vi "Initialization VI.vi"(8 "error in (no error)":errorcluster, 10 "Custom XML":string, 11 "Device Item Ref in":T1 format="%.0x") -> (0 "error out":errorcluster, 3 "Device Item Ref out":T1 format="%.0x")   [LabVIEW 2019, in "Protection and Counter Addon System Explorer.lvlib"]
uses:
  Protection and Counter Addon System Explorer.lvlib
  <vilib>/NI VeriStand/Custom Device API/Custom Device Item Ref.ctl
  <vilib>/NI VeriStand/Custom Device API/Custom Device Channel.ctl
  <vilib>/NI VeriStand/Custom Device API/Custom Device Channel Type.ctl
  Addon Shared/SubVIs/GUID Lookup.vi
  <vilib>/NI VeriStand/Custom Device API/Custom Device API.lvlib
  Addon Shared/Protection and Counter Addon Shared.lvlib
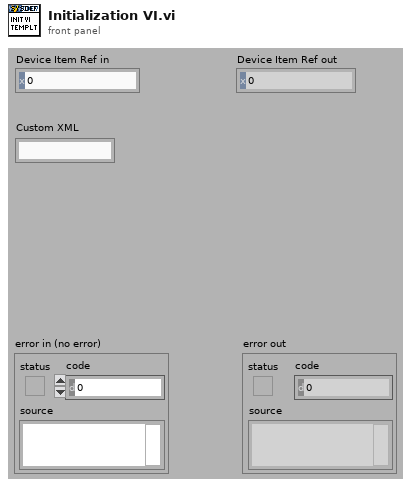
[diagram p1: front panel]
types:
  T1 = typedef "Custom Device API.lvlib/Custom Device Item Ref.ctl" = u64
  T2 = typedef "Custom Device API.lvlib/Custom Device Channel.ctl" = cluster{"Type":T3, "Units":string, "Default Value":dbl, "Faultable":bool, "Scalable":bool}
  T3 = typedef "Custom Device API.lvlib/Custom Device Channel Type.ctl" = enum16{"Input", "Output"}
  T4 = typedef "Protection and Counter Addon Shared.lvlib/XNET Settings.ctl" = cluster{"Database":refnum<k21>, "Cluster":refnum<k21>, "Port":string, "Baud rate [Bd]":u64, "Termination":u32, "CAN I/O Mode":u32, "FD Baud rate [Bd]":u64, "Priority":i32, "Use Legacy":bool}
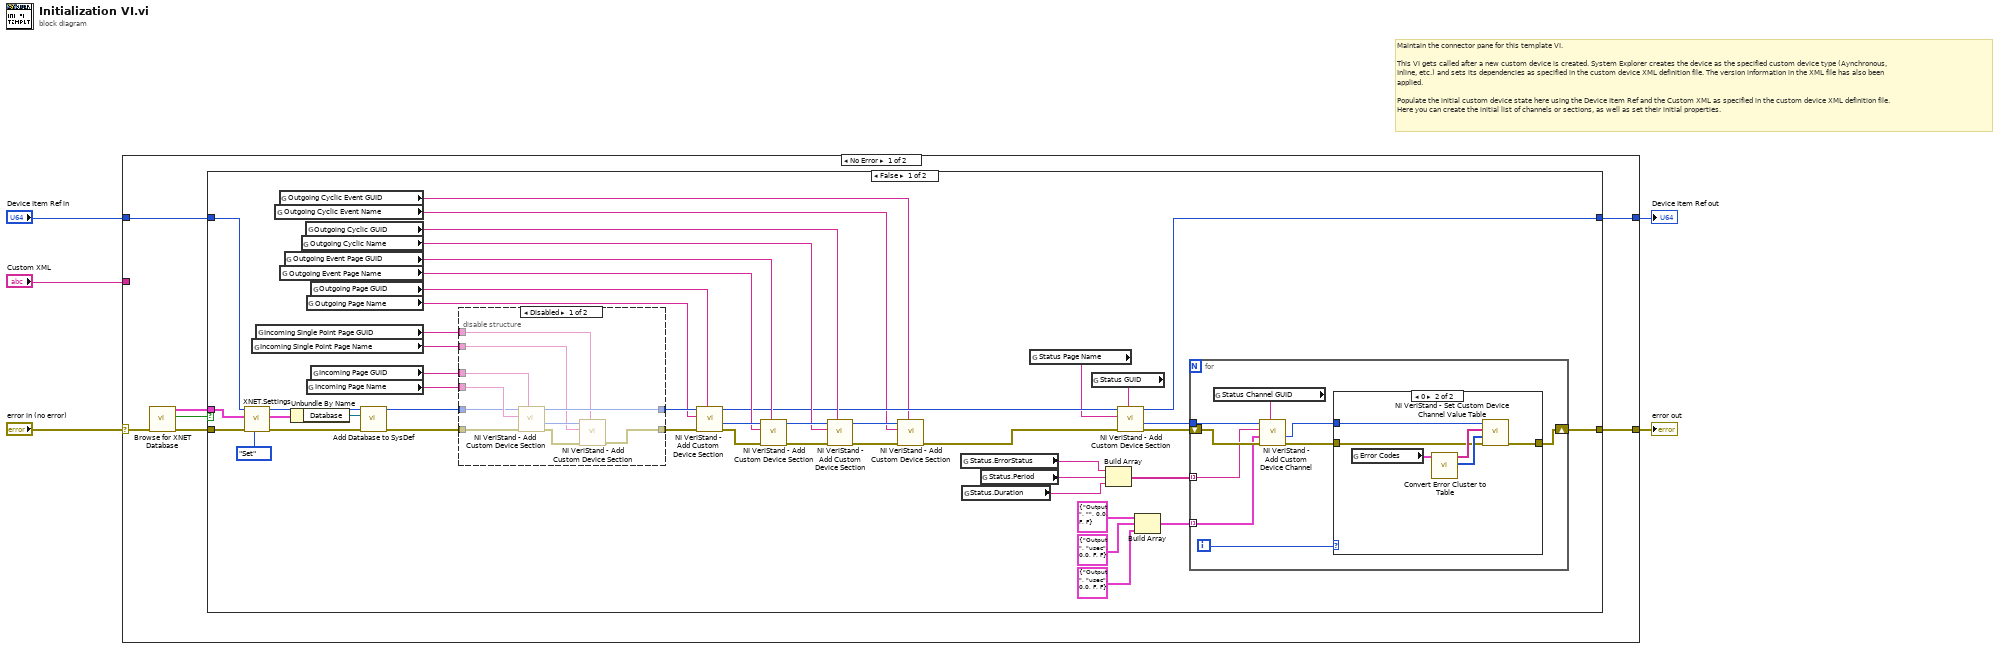
[diagram p0: block diagram]
diagram:
  # "Maintain the connector pane for this template VI.\n\nThis VI gets called after a new custom device is created. System Explorer creates the device as the specified custom device type (Aynchronous, Inline, etc.) and sets its dependencies as specified in the custom device XML definition file. The version information in the XML file has also been applied.\n\nPopulate the initial custom device state here using the Device Item Ref and the Custom XML as specified in the custom device XML definition file. Here you can create the initial list of channels or sections, as well as set their initial properties."
  n1 = case shown="No Error" "error in (no error)" {
    selector: "error in (no error)" -> [w10 w90]
    tunnel: [w12 w90] -> w5
    tunnel: [w11 w89] -> w3
    tunnel: "Device Item Ref in" -> [w8 w89]
    tunnel: "Custom XML" -> [_ _]
    frame No Error {
      n2 = call "Browse for XNET Database.vi"("error in (no error)"=w10) -> ("error out"=w9:errorcluster, "Cancel Out"=w7:bool, "XNET Settings"=w6:T4)  [unwired: 8 in]
      n3 = case shown="False" w7 {
        tunnel: [w28 w88] -> w12
        tunnel: [w29 w87] -> w11
        tunnel: w9 -> [w51 w88]
        tunnel: w8 -> [w49 w87]
        tunnel: w6 -> [w47 _]
        frame False {
          n4 = call "XNET.Settings.vi"("Action"=enum8{"Get", "Set"}."Set", "error in (no error)"=w51, "XNET Settings"=w47, "Parent Ref in"=w49) -> ("error out"=w50:errorcluster, "XNET Settings"=w46:T4, "Item Ref out"=w48:T1)  [unwired: 5 in]
          n5 = global read "GUID Lookup.vi" "Incoming Single Point Page Name"() -> (w33:string)
          n6 = global read "GUID Lookup.vi" "Incoming Single Point Page GUID"() -> (w34:string)
          n7 = global read "GUID Lookup.vi" "Outgoing Cyclic Event Name"() -> (w17:string)
          n8 = global read "GUID Lookup.vi" "Outgoing Cyclic Event GUID"() -> (w18:string)
          n9 = global read "GUID Lookup.vi" "Outgoing Event Page Name"() -> (w38:string)
          n10 = global read "GUID Lookup.vi" "Outgoing Event Page GUID"() -> (w39:string)
          n11 = Unbundle By Name(w46) -> ("Database"=w45:refnum<k21>)
          n12 = global read "GUID Lookup.vi" "Outgoing Cyclic Name"() -> (w36:string)
          n13 = global read "GUID Lookup.vi" "Outgoing Cyclic GUID"() -> (w37:string)
          n14 = global read "GUID Lookup.vi" "Outgoing Page Name"() -> (w55:string)
          n15 = global read "GUID Lookup.vi" "Incoming Page Name"() -> (w54:string)
          n16 = global read "GUID Lookup.vi" "Outgoing Page GUID"() -> (w56:string)
          n17 = global read "GUID Lookup.vi" "Incoming Page GUID"() -> (w58:string)
          n18 = call "Add Database to SysDef.vi"("error in"=w50, "DB Alias"=w45, "Item Ref in"=w48) -> ("error out"=w53:errorcluster, "Item Ref out"=w52:T1)  [unwired: 7 in]
          n19 = disable-structure shown="Disabled" {
            disable-tunnel: w58 -> [w84 _]
            disable-tunnel: [w83 w85] -> w57
            disable-tunnel: w54 -> [w82 _]
            disable-tunnel: w53 -> [w81 w86]
            disable-tunnel: w52 -> [w80 w85]
            disable-tunnel: [w77 w86] -> w35
            disable-tunnel: w34 -> [w76 _]
            disable-tunnel: w33 -> [w75 _]
            frame Disabled {
              n20 = call <vilib>:"NI VeriStand - Add Custom Device Section.vi"("GUID (Default Section)"=w84, "error in (no error)"=w81, "Section Name"=w82, "Parent Ref in"=w80) -> ("error out"=w78:errorcluster, "Section Ptr"=w79:T1, "Parent Ref out"=w83:T1)  [unwired: 4 in, 1 out]
              n21 = call <vilib>:"NI VeriStand - Add Custom Device Section.vi"("GUID (Default Section)"=w76, "error in (no error)"=w78, "Section Name"=w75, "Parent Ref in"=w79) -> ("error out"=w77:errorcluster)  [unwired: 4 in, 3 out]
            }
            frame Enabled {
            }
          }
          n22 = call <vilib>:"NI VeriStand - Add Custom Device Section.vi"("GUID (Default Section)"=w56, "error in (no error)"=w35, "Section Name"=w55, "Parent Ref in"=w57) -> ("error out"=w41:errorcluster, "Section Ptr"=w43:T1, "Parent Ref out"=w30:T1)  [unwired: 4 in, 1 out]
          n23 = call <vilib>:"NI VeriStand - Add Custom Device Section.vi"("GUID (Default Section)"=w39, "error in (no error)"=w41, "Section Name"=w38, "Parent Ref in"=w43) -> ("error out"=w42:errorcluster, "Parent Ref out"=w40:T1)  [unwired: 4 in, 2 out]
          n24 = call <vilib>:"NI VeriStand - Add Custom Device Section.vi"("GUID (Default Section)"=w37, "error in (no error)"=w42, "Section Name"=w36, "Parent Ref in"=w40) -> ("error out"=w20:errorcluster, "Parent Ref out"=w21:T1)  [unwired: 4 in, 2 out]
          n25 = call <vilib>:"NI VeriStand - Add Custom Device Section.vi"("GUID (Default Section)"=w18, "error in (no error)"=w20, "Section Name"=w17, "Parent Ref in"=w21) -> ("error out"=w19:errorcluster)  [unwired: 4 in, 3 out]
          n26 = global read "GUID Lookup.vi" "Status.ErrorStatus"() -> (w27:string)
          n27 = global read "GUID Lookup.vi" "Status.Duration"() -> (w25:string)
          n28 = global read "GUID Lookup.vi" "Status.Period"() -> (w26:string)
          n29 = global read "GUID Lookup.vi" "Status Page Name"() -> (w22:string)
          n30 = global read "GUID Lookup.vi" "Status GUID"() -> (w23:string)
          n31 = Build Array(w27, w26, w25) -> (w24:string[])
          n32 = call <vilib>:"NI VeriStand - Add Custom Device Section.vi"("GUID (Default Section)"=w23, "error in (no error)"=w19, "Section Name"=w22, "Parent Ref in"=w30) -> ("error out"=w31:errorcluster, "Section Ptr"=w32:T1, "Parent Ref out"=w29:T1)  [unwired: 4 in, 1 out]
          n33 = Build Array(T2 {"Type"=enum."Output", "Units"="", "Default Value"=0.0, "Faultable"=FALSE, "Scalable"=FALSE} ("Channel"), T2 {"Type"=enum."Output", "Units"="usec", "Default Value"=0.0, "Faultable"=FALSE, "Scalable"=FALSE} ("Channel"), T2 {"Type"=enum."Output", "Units"="usec", "Default Value"=0.0, "Faultable"=FALSE, "Scalable"=FALSE} ("Channel")) -> (w13:T2[])
          n34 = for {
            tunnel: w32 -> [w67]
            shift-right: [w60] -> w28
            shift-left: w31 -> [w66]
            tunnel: w24 -> [w64] mode=indexing
            tunnel: w13 -> [w63] mode=indexing
            i -> [w62]
            n35 = global read "GUID Lookup.vi" "Status Channel GUID"() -> (w65:string)
            n36 = call <vilib>:"NI VeriStand - Add Custom Device Channel.vi"("GUID (Default Channel)"=w65, "error in (no error)"=w66, "Channel"=w63, "Channel Name"=w64, "Parent Ref in"=w67) -> ("error out"=w61:errorcluster, "Channel Ref"=w59:T1)  [unwired: 3 in, 2 out]
            n37 = case shown="0" w62 {
              tunnel: w59 -> [_ w73]
              tunnel: w61 -> [w68 w70]
              tunnel: [w68 w69] -> w60
              frame Default {
              }
              frame 0 {
                n38 = global read "GUID Lookup.vi" "Error Codes"() -> (w74:cluster{"number":i32, "trimmed string":string}[])
                n39 = call "Convert Error Cluster to Table.vi"("Error Codes"=w74) -> ("Code"=w71:i32[], "String"=w72:string[])  [unwired: 9 in]
                n40 = call <vilib>:"NI VeriStand - Set Custom Device Channel Value Table.vi"("error in (no error)"=w70, "Values"=w71, "Names"=w72, "Channel Ref in"=w73) -> ("error out"=w69:errorcluster)  [unwired: 6 in, 1 out]
              }
            }
          }
        }
        frame True {
        }
      }
    }
    frame Error {
    }
  }
  "error out" <- w5
  "Device Item Ref out" <- w3
